vi "Set Worker Functions.vi"(8 "error in (no error)":errorcluster, 9 "Functions":string[](array[string]), 10 "Name":string, 11 "Application Controller in":refnum<class "Application Controller.lvclass">) -> (0 "error out":errorcluster, 3 "Application Controller out":refnum<class "Application Controller.lvclass">)   [LabVIEW 2016, in "Application Controller.lvclass"]
uses:
  Application Controller.lvclass
  Application Controller.lvclass/Application Controller.ctl
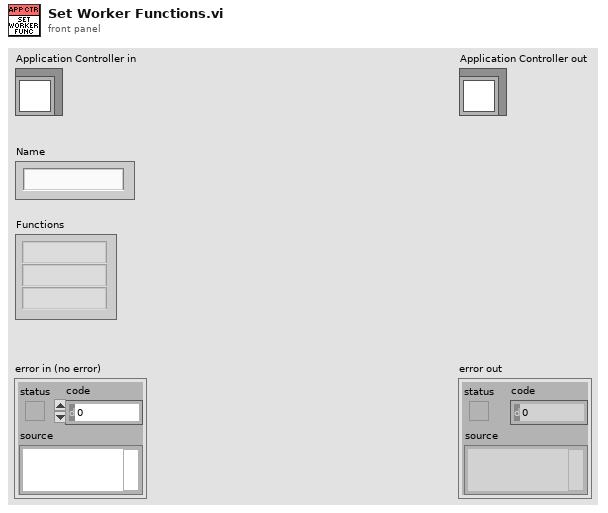
[diagram p1: front panel]
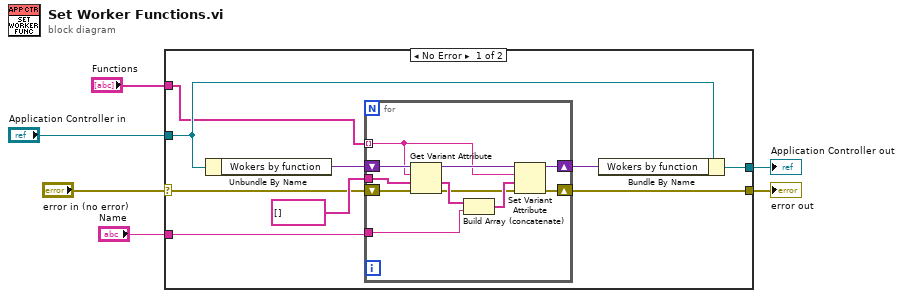
[diagram p0: block diagram]
diagram:
  n1 = case shown="No Error" "error in (no error)" {
    selector: "error in (no error)" -> [w8 w28]
    tunnel: [w7 w28] -> w5
    tunnel: [w10 w27] -> w3
    tunnel: "Application Controller in" -> [w15 w27]
    tunnel: "Functions" -> [w14 _]
    tunnel: "Name" -> [w11 _]
    frame No Error {
      n2 = Unbundle By Name(w15) -> ("Wokers by function"=w13:variant)
      n3 = for {
        tunnel: w14 -> [w20] mode=indexing
        tunnel: string[] [] -> [w25]
        shift-right: [w22] -> w9
        shift-left: w13 -> [w26]
        tunnel: w11 -> [w21]
        shift-right: [w17] -> w7
        shift-left: w8 -> [w16]
        n4 = Get Variant Attribute(Variant=w26, name=w20, default value (empty Variant)=w25, error in=w16) -> (duplicate Variant=w23:variant, value=w24:string[], error out=w18:errorcluster)  [unwired: 1 out]
        n5 = Build Array (concatenate)(w24, w21) -> (w19:string[])
        n6 = Set Variant Attribute(Variant=w23, name=w20, value=w19, error in=w18) -> (Variant out=w22:variant, error out=w17:errorcluster)  [unwired: 1 out]
      }
      n7 = Bundle By Name(cluster=w15, "Wokers by function"=w9) -> (w10:refnum<class "Application Controller.lvclass">)
    }
    frame Error {
    }
  }
  "error out" <- w5
  "Application Controller out" <- w3
